vi "readLogHardpointActuatorInfo.vi"(8 "error in (no error)":errorcluster, 10 "Parser":refnum<class "U8ArrayParserAutoIndexing.lvclass">, 11 "M1M3SAL in":refnum<class "M1M3SAL.lvclass">) -> (0 "error out":errorcluster, 2 "EventHardpointActuatorInfo":variant, 3 "M1M3SAL out":refnum<class "M1M3SAL.lvclass">)   [LabVIEW 2016, in "M1M3SupportCommunicator.lvlib" / "M1M3SAL.lvclass"]
uses:
  M1M3SAL.lvclass
  Common_RT_Utilities/U8ArrayParserAutoIndexing/U8ArrayParserAutoIndexing.lvclass
  DataTypes/Topics/EventHardpointActuatorInfo.ctl
  DataTypes/Topics/Parts/Timestamp.ctl
  DataTypes/Topics/M1M3SupportTopics.lvlib
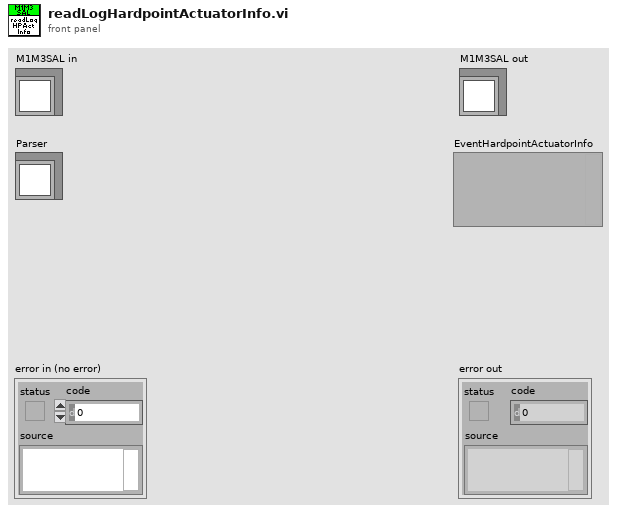
[diagram p1: front panel]
types:
  T1 = typedef "M1M3SupportTopics.lvlib/EventHardpointActuatorInfo.ctl" = cluster{"Timestamp":T2, "ReferenceId":i32[], "ReferencePosition":i32[], "XPosition":sgl[], "YPosition":sgl[], "ZPosition":sgl[], "ILCUniqueId":i64[], "ILCApplicationType":u8[], "NetworkNodeType":u8[], "ILCSelectedOptions":u8[], "NetworkNodeOptions":u8[], "MajorRevision":u8[], "MinorRevision":u8[], "ADCScanRate":u8[], "MainADCCalibrationK1":sgl[], "MainADCCalibrationK2":sgl[], "MainADCCalibrationK3":sgl[], "MainADCCalibrationK4":sgl[], "MainLoadCellOffset":sgl[], "MainLoadCellSensitivity":sgl[], "BackupADCCalibrationK1":sgl[], "BackupADCCalibrationK2":sgl[], "BackupADCCalibrationK3":sgl[], "BackupADCCalibrationK4":sgl[], "BackupLoadCellOffset":sgl[], "BackupLoadCellSensitivity":sgl[], "MainCalibrationError":bool[], "BackupCalibrationError":bool[], "UniqueIdCRCError":bool[], "ApplicationTypeMismatch":bool[], "ApplicationMissing":bool[], "ApplicationCRCMismatch":bool[], "OneWireMissing":bool[], "OneWire1Mismatch":bool[], "OneWire2Mismatch":bool[]}
  T2 = typedef "M1M3SupportTopics.lvlib/Timestamp.ctl" = dbl
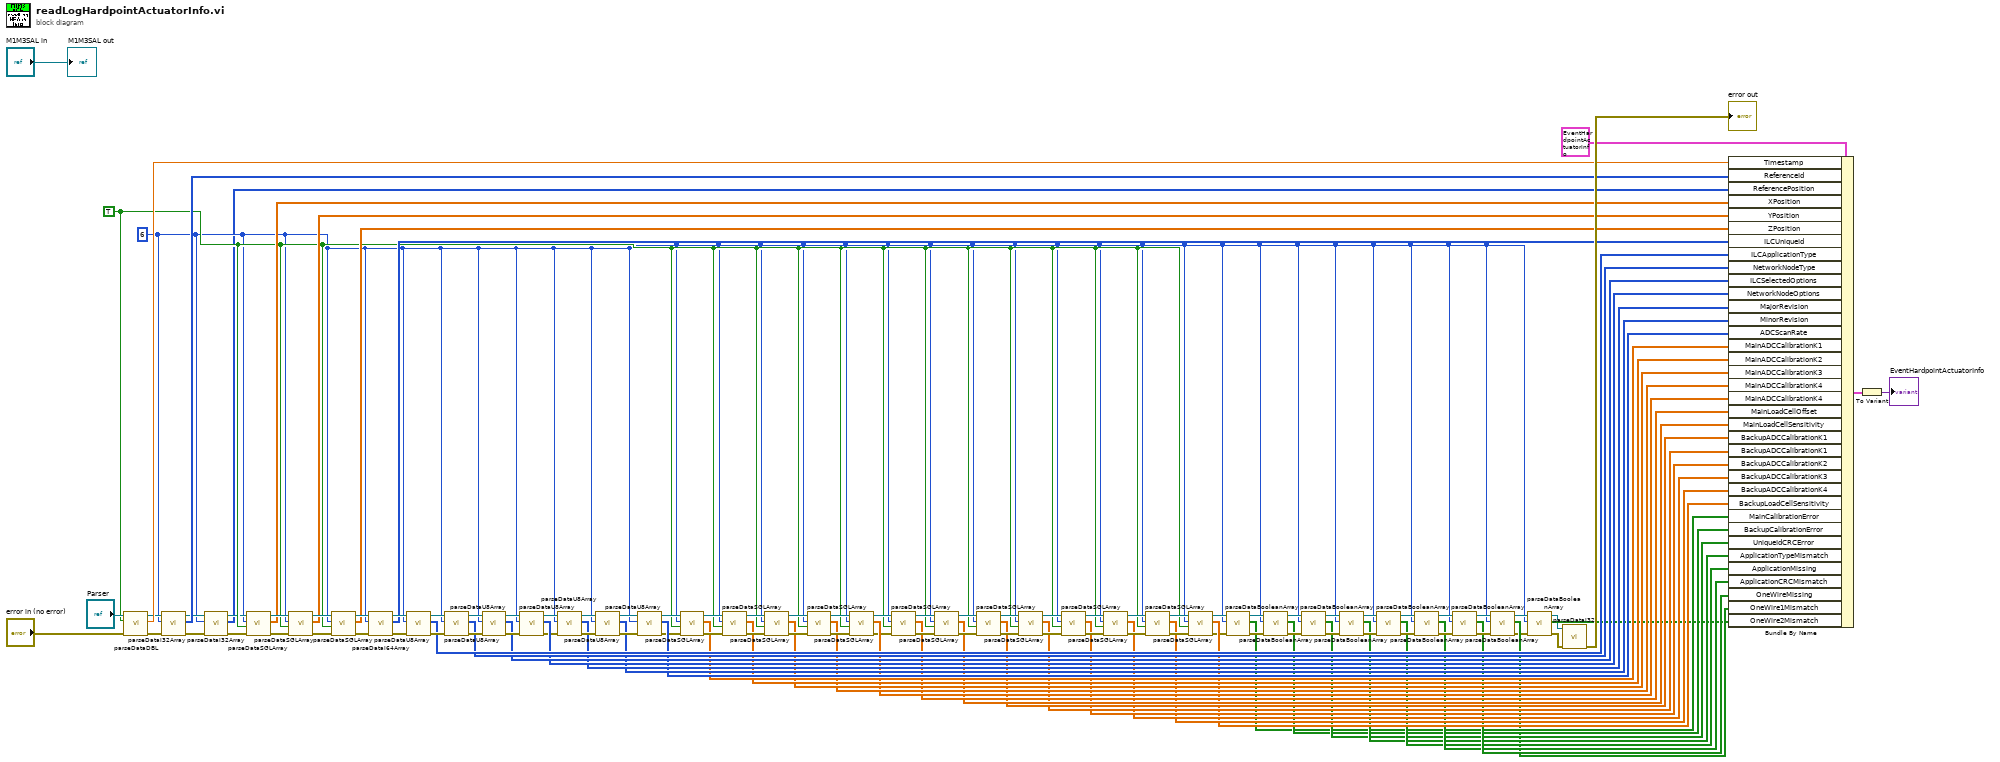
[diagram p0: block diagram]
diagram:
  w4 = 6
  w37 = TRUE ("OverrideSwapBytes")
  n1 = call "parseDataDBL.vi"("error in (no error)"="error in (no error)", "OverrideSwapBytes"=w37, "U8ArrayParserAutoIndexing in"="Parser") -> ("error out"=w38:errorcluster, "Data"=w111:dbl, "U8ArrayParserAutoIndexing out"=w39:refnum<class "U8ArrayParserAutoIndexing.lvclass">)  [unwired: 6 in]
  n2 = call "parseDataI32Array.vi"("U8ArrayParserAutoIndexing in"=w39, "Length"=w4, "error in (no error)"=w38) -> ("U8ArrayParserAutoIndexing out"=w8:refnum<class "U8ArrayParserAutoIndexing.lvclass">, "Data"=w96:i32[], "error out"=w5:errorcluster)  [unwired: 5 in]
  n3 = call "parseDataI32Array.vi"("U8ArrayParserAutoIndexing in"=w8, "Length"=w4, "error in (no error)"=w5) -> ("U8ArrayParserAutoIndexing out"=w7:refnum<class "U8ArrayParserAutoIndexing.lvclass">, "Data"=w3:i32[], "error out"=w6:errorcluster)  [unwired: 5 in]
  n4 = call "parseDataSGLArray.vi"("U8ArrayParserAutoIndexing in"=w7, "Length"=w4, "OverrideSwapBytes"=w37, "error in (no error)"=w6) -> ("U8ArrayParserAutoIndexing out"=w110:refnum<class "U8ArrayParserAutoIndexing.lvclass">, "Data"=w95:sgl[], "error out"=w109:errorcluster)  [unwired: 4 in]
  n5 = call "parseDataSGLArray.vi"("U8ArrayParserAutoIndexing in"=w110, "Length"=w4, "OverrideSwapBytes"=w37, "error in (no error)"=w109) -> ("U8ArrayParserAutoIndexing out"=w108:refnum<class "U8ArrayParserAutoIndexing.lvclass">, "Data"=w94:sgl[], "error out"=w107:errorcluster)  [unwired: 4 in]
  n6 = call "parseDataSGLArray.vi"("U8ArrayParserAutoIndexing in"=w108, "Length"=w4, "OverrideSwapBytes"=w37, "error in (no error)"=w107) -> ("U8ArrayParserAutoIndexing out"=w106:refnum<class "U8ArrayParserAutoIndexing.lvclass">, "Data"=w93:sgl[], "error out"=w105:errorcluster)  [unwired: 4 in]
  n7 = call "parseDataI64Array.vi"("U8ArrayParserAutoIndexing in"=w106, "Length"=w4, "error in (no error)"=w105) -> ("U8ArrayParserAutoIndexing out"=w104:refnum<class "U8ArrayParserAutoIndexing.lvclass">, "Data"=w92:i64[], "error out"=w103:errorcluster)  [unwired: 5 in]
  n8 = call "parseDataU8Array.vi"("U8ArrayParserAutoIndexing in"=w104, "Length"=w4, "error in (no error)"=w103) -> ("U8ArrayParserAutoIndexing out"=w102:refnum<class "U8ArrayParserAutoIndexing.lvclass">, "Data"=w91:u8[], "error out"=w101:errorcluster)  [unwired: 5 in]
  n9 = call "parseDataU8Array.vi"("U8ArrayParserAutoIndexing in"=w102, "Length"=w4, "error in (no error)"=w101) -> ("U8ArrayParserAutoIndexing out"=w100:refnum<class "U8ArrayParserAutoIndexing.lvclass">, "Data"=w90:u8[], "error out"=w99:errorcluster)  [unwired: 5 in]
  n10 = call "parseDataU8Array.vi"("U8ArrayParserAutoIndexing in"=w100, "Length"=w4, "error in (no error)"=w99) -> ("U8ArrayParserAutoIndexing out"=w98:refnum<class "U8ArrayParserAutoIndexing.lvclass">, "Data"=w89:u8[], "error out"=w97:errorcluster)  [unwired: 5 in]
  n11 = call "parseDataU8Array.vi"("U8ArrayParserAutoIndexing in"=w98, "Length"=w4, "error in (no error)"=w97) -> ("U8ArrayParserAutoIndexing out"=w65:refnum<class "U8ArrayParserAutoIndexing.lvclass">, "Data"=w88:u8[], "error out"=w64:errorcluster)  [unwired: 5 in]
  n12 = call "parseDataU8Array.vi"("U8ArrayParserAutoIndexing in"=w65, "Length"=w4, "error in (no error)"=w64) -> ("U8ArrayParserAutoIndexing out"=w87:refnum<class "U8ArrayParserAutoIndexing.lvclass">, "Data"=w83:u8[], "error out"=w86:errorcluster)  [unwired: 5 in]
  n13 = call "parseDataU8Array.vi"("U8ArrayParserAutoIndexing in"=w87, "Length"=w4, "error in (no error)"=w86) -> ("U8ArrayParserAutoIndexing out"=w85:refnum<class "U8ArrayParserAutoIndexing.lvclass">, "Data"=w82:u8[], "error out"=w84:errorcluster)  [unwired: 5 in]
  n14 = call "parseDataU8Array.vi"("U8ArrayParserAutoIndexing in"=w85, "Length"=w4, "error in (no error)"=w84) -> ("U8ArrayParserAutoIndexing out"=w80:refnum<class "U8ArrayParserAutoIndexing.lvclass">, "Data"=w81:u8[], "error out"=w79:errorcluster)  [unwired: 5 in]
  n15 = call "parseDataSGLArray.vi"("U8ArrayParserAutoIndexing in"=w80, "Length"=w4, "OverrideSwapBytes"=w37, "error in (no error)"=w79) -> ("U8ArrayParserAutoIndexing out"=w76:refnum<class "U8ArrayParserAutoIndexing.lvclass">, "Data"=w70:sgl[], "error out"=w75:errorcluster)  [unwired: 4 in]
  n16 = call "parseDataSGLArray.vi"("U8ArrayParserAutoIndexing in"=w76, "Length"=w4, "OverrideSwapBytes"=w37, "error in (no error)"=w75) -> ("U8ArrayParserAutoIndexing out"=w78:refnum<class "U8ArrayParserAutoIndexing.lvclass">, "Data"=w69:sgl[], "error out"=w77:errorcluster)  [unwired: 4 in]
  n17 = call "parseDataSGLArray.vi"("U8ArrayParserAutoIndexing in"=w78, "Length"=w4, "OverrideSwapBytes"=w37, "error in (no error)"=w77) -> ("U8ArrayParserAutoIndexing out"=w74:refnum<class "U8ArrayParserAutoIndexing.lvclass">, "Data"=w68:sgl[], "error out"=w73:errorcluster)  [unwired: 4 in]
  n18 = call "parseDataSGLArray.vi"("U8ArrayParserAutoIndexing in"=w74, "Length"=w4, "OverrideSwapBytes"=w37, "error in (no error)"=w73) -> ("U8ArrayParserAutoIndexing out"=w72:refnum<class "U8ArrayParserAutoIndexing.lvclass">, "Data"=w67:sgl[], "error out"=w71:errorcluster)  [unwired: 4 in]
  n19 = call "parseDataSGLArray.vi"("U8ArrayParserAutoIndexing in"=w72, "Length"=w4, "OverrideSwapBytes"=w37, "error in (no error)"=w71) -> ("U8ArrayParserAutoIndexing out"=w41:refnum<class "U8ArrayParserAutoIndexing.lvclass">, "Data"=w66:sgl[], "error out"=w40:errorcluster)  [unwired: 4 in]
  n20 = call "parseDataSGLArray.vi"("U8ArrayParserAutoIndexing in"=w41, "Length"=w4, "OverrideSwapBytes"=w37, "error in (no error)"=w40) -> ("U8ArrayParserAutoIndexing out"=w63:refnum<class "U8ArrayParserAutoIndexing.lvclass">, "Data"=w49:sgl[], "error out"=w62:errorcluster)  [unwired: 4 in]
  n21 = call "parseDataSGLArray.vi"("U8ArrayParserAutoIndexing in"=w63, "Length"=w4, "OverrideSwapBytes"=w37, "error in (no error)"=w62) -> ("U8ArrayParserAutoIndexing out"=w61:refnum<class "U8ArrayParserAutoIndexing.lvclass">, "Data"=w48:sgl[], "error out"=w60:errorcluster)  [unwired: 4 in]
  n22 = call "parseDataSGLArray.vi"("U8ArrayParserAutoIndexing in"=w61, "Length"=w4, "OverrideSwapBytes"=w37, "error in (no error)"=w60) -> ("U8ArrayParserAutoIndexing out"=w59:refnum<class "U8ArrayParserAutoIndexing.lvclass">, "Data"=w47:sgl[], "error out"=w58:errorcluster)  [unwired: 4 in]
  n23 = call "parseDataSGLArray.vi"("U8ArrayParserAutoIndexing in"=w59, "Length"=w4, "OverrideSwapBytes"=w37, "error in (no error)"=w58) -> ("U8ArrayParserAutoIndexing out"=w57:refnum<class "U8ArrayParserAutoIndexing.lvclass">, "Data"=w46:sgl[], "error out"=w56:errorcluster)  [unwired: 4 in]
  n24 = call "parseDataSGLArray.vi"("U8ArrayParserAutoIndexing in"=w57, "Length"=w4, "OverrideSwapBytes"=w37, "error in (no error)"=w56) -> ("U8ArrayParserAutoIndexing out"=w55:refnum<class "U8ArrayParserAutoIndexing.lvclass">, "Data"=w45:sgl[], "error out"=w54:errorcluster)  [unwired: 4 in]
  n25 = call "parseDataSGLArray.vi"("U8ArrayParserAutoIndexing in"=w55, "Length"=w4, "OverrideSwapBytes"=w37, "error in (no error)"=w54) -> ("U8ArrayParserAutoIndexing out"=w53:refnum<class "U8ArrayParserAutoIndexing.lvclass">, "Data"=w44:sgl[], "error out"=w52:errorcluster)  [unwired: 4 in]
  n26 = call "parseDataSGLArray.vi"("U8ArrayParserAutoIndexing in"=w53, "Length"=w4, "OverrideSwapBytes"=w37, "error in (no error)"=w52) -> ("U8ArrayParserAutoIndexing out"=w51:refnum<class "U8ArrayParserAutoIndexing.lvclass">, "Data"=w43:sgl[], "error out"=w50:errorcluster)  [unwired: 4 in]
  n27 = call "parseDataSGLArray.vi"("U8ArrayParserAutoIndexing in"=w51, "Length"=w4, "OverrideSwapBytes"=w37, "error in (no error)"=w50) -> ("U8ArrayParserAutoIndexing out"=w34:refnum<class "U8ArrayParserAutoIndexing.lvclass">, "Data"=w42:sgl[], "error out"=w35:errorcluster)  [unwired: 4 in]
  n28 = call "parseDataBooleanArray.vi"("error in (no error)"=w35, "Length"=w4, "U8ArrayParserAutoIndexing in"=w34) -> ("error out"=w33:errorcluster, "Data"=w13:bool[], "U8ArrayParserAutoIndexing out"=w32:refnum<class "U8ArrayParserAutoIndexing.lvclass">)  [unwired: 6 in]
  n29 = call "parseDataBooleanArray.vi"("error in (no error)"=w33, "Length"=w4, "U8ArrayParserAutoIndexing in"=w32) -> ("error out"=w31:errorcluster, "Data"=w14:bool[], "U8ArrayParserAutoIndexing out"=w30:refnum<class "U8ArrayParserAutoIndexing.lvclass">)  [unwired: 6 in]
  n30 = call "parseDataBooleanArray.vi"("error in (no error)"=w31, "Length"=w4, "U8ArrayParserAutoIndexing in"=w30) -> ("error out"=w29:errorcluster, "Data"=w15:bool[], "U8ArrayParserAutoIndexing out"=w28:refnum<class "U8ArrayParserAutoIndexing.lvclass">)  [unwired: 6 in]
  n31 = call "parseDataBooleanArray.vi"("error in (no error)"=w29, "Length"=w4, "U8ArrayParserAutoIndexing in"=w28) -> ("error out"=w27:errorcluster, "Data"=w16:bool[], "U8ArrayParserAutoIndexing out"=w26:refnum<class "U8ArrayParserAutoIndexing.lvclass">)  [unwired: 6 in]
  n32 = call "parseDataBooleanArray.vi"("error in (no error)"=w27, "Length"=w4, "U8ArrayParserAutoIndexing in"=w26) -> ("error out"=w25:errorcluster, "Data"=w17:bool[], "U8ArrayParserAutoIndexing out"=w24:refnum<class "U8ArrayParserAutoIndexing.lvclass">)  [unwired: 6 in]
  n33 = call "parseDataBooleanArray.vi"("error in (no error)"=w25, "Length"=w4, "U8ArrayParserAutoIndexing in"=w24) -> ("error out"=w23:errorcluster, "Data"=w18:bool[], "U8ArrayParserAutoIndexing out"=w22:refnum<class "U8ArrayParserAutoIndexing.lvclass">)  [unwired: 6 in]
  n34 = call "parseDataBooleanArray.vi"("error in (no error)"=w23, "Length"=w4, "U8ArrayParserAutoIndexing in"=w22) -> ("error out"=w20:errorcluster, "Data"=w19:bool[], "U8ArrayParserAutoIndexing out"=w21:refnum<class "U8ArrayParserAutoIndexing.lvclass">)  [unwired: 6 in]
  n35 = call "parseDataBooleanArray.vi"("error in (no error)"=w20, "Length"=w4, "U8ArrayParserAutoIndexing in"=w21) -> ("error out"=w10:errorcluster, "Data"=w12:bool[], "U8ArrayParserAutoIndexing out"=w11:refnum<class "U8ArrayParserAutoIndexing.lvclass">)  [unwired: 6 in]
  n36 = call "parseDataBooleanArray.vi"("error in (no error)"=w10, "Length"=w4, "U8ArrayParserAutoIndexing in"=w11) -> ("error out"=w1:errorcluster, "Data"=w9:bool[], "U8ArrayParserAutoIndexing out"=w2:refnum<class "U8ArrayParserAutoIndexing.lvclass">)  [unwired: 6 in]
  n37 = call "parseDataI32.vi"("error in (no error)"=w1, "U8ArrayParserAutoIndexing in"=w2) -> ("error out"=→"error out":errorcluster)  [unwired: 7 in, 2 out]
  n38 = Bundle By Name(cluster=T1 {"Timestamp"=0.0, "ReferenceId"=[], "ReferencePosition"=[], "XPosition"=[], "YPosition"=[], "ZPosition"=[], "ILCUniqueId"=[], "ILCApplicationType"=[], "NetworkNodeType"=[], "ILCSelectedOptions"=[], "NetworkNodeOptions"=[], "MajorRevision"=[], "MinorRevision"=[], "ADCScanRate"=[], "MainADCCalibrationK1"=[], "MainADCCalibrationK2"=[], "MainADCCalibrationK3"=[], "MainADCCalibrationK4"=[], "MainLoadCellOffset"=[], "MainLoadCellSensitivity"=[], "BackupADCCalibrationK1"=[], "BackupADCCalibrationK2"=[], "BackupADCCalibrationK3"=[], "BackupADCCalibrationK4"=[], "BackupLoadCellOffset"=[], "BackupLoadCellSensitivity"=[], "MainCalibrationError"=[], "BackupCalibrationError"=[], "UniqueIdCRCError"=[], "ApplicationTypeMismatch"=[], "ApplicationMissing"=[], "ApplicationCRCMismatch"=[], "OneWireMissing"=[], "OneWire1Mismatch"=[], "OneWire2Mismatch"=[]} ("EventHardpointActuatorInfo"), "Timestamp"=w111, "ReferenceId"=w96, "ReferencePosition"=w3, "XPosition"=w95, "YPosition"=w94, "ZPosition"=w93, "ILCUniqueId"=w92, "ILCApplicationType"=w91, "NetworkNodeType"=w90, "ILCSelectedOptions"=w89, "NetworkNodeOptions"=w88, "MajorRevision"=w83, "MinorRevision"=w82, "ADCScanRate"=w81, "MainADCCalibrationK1"=w70, "MainADCCalibrationK2"=w69, "MainADCCalibrationK3"=w68, "MainADCCalibrationK4"=w67, "MainADCCalibrationK4"=w66, "MainLoadCellOffset"=w49, "MainLoadCellSensitivity"=w48, "BackupADCCalibrationK1"=w47, "BackupADCCalibrationK1"=w46, "BackupADCCalibrationK2"=w45, "BackupADCCalibrationK3"=w44, "BackupADCCalibrationK4"=w43, "BackupLoadCellSensitivity"=w42, "MainCalibrationError"=w13, "BackupCalibrationError"=w14, "UniqueIdCRCError"=w15, "ApplicationTypeMismatch"=w16, "ApplicationMissing"=w17, "ApplicationCRCMismatch"=w18, "OneWireMissing"=w19, "OneWire1Mismatch"=w12, "OneWire2Mismatch"=w9) -> (w116:T1)
  n39 = To Variant(anything=w116) -> (Variant=→"EventHardpointActuatorInfo":variant)
  "M1M3SAL out" <- "M1M3SAL in"
